vi "alignTop.vi"(6 "useControlBodyOnly":bool, 8 "error in (no error)":errorcluster, 11 "refs":refnum<vi>[](array[refnum])) -> (0 "error out":errorcluster, 3 "refs(dup)":refnum<vi>[](array[refnum]))   [LabVIEW 2023, in "TLC_Geometry.lvlib"]
doc: "Aligns all controls to the topmost position among the input controls.\nThe topmost coordinate is computed and applied to all controls."
uses:
  TLC_Geometry.lvlib
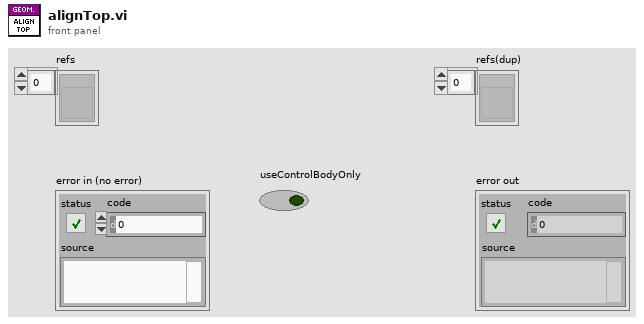
[diagram p1: front panel]
types:
  T1 = cluster{"left":i32, "top":i32, "right":i32, "bottom":i32}
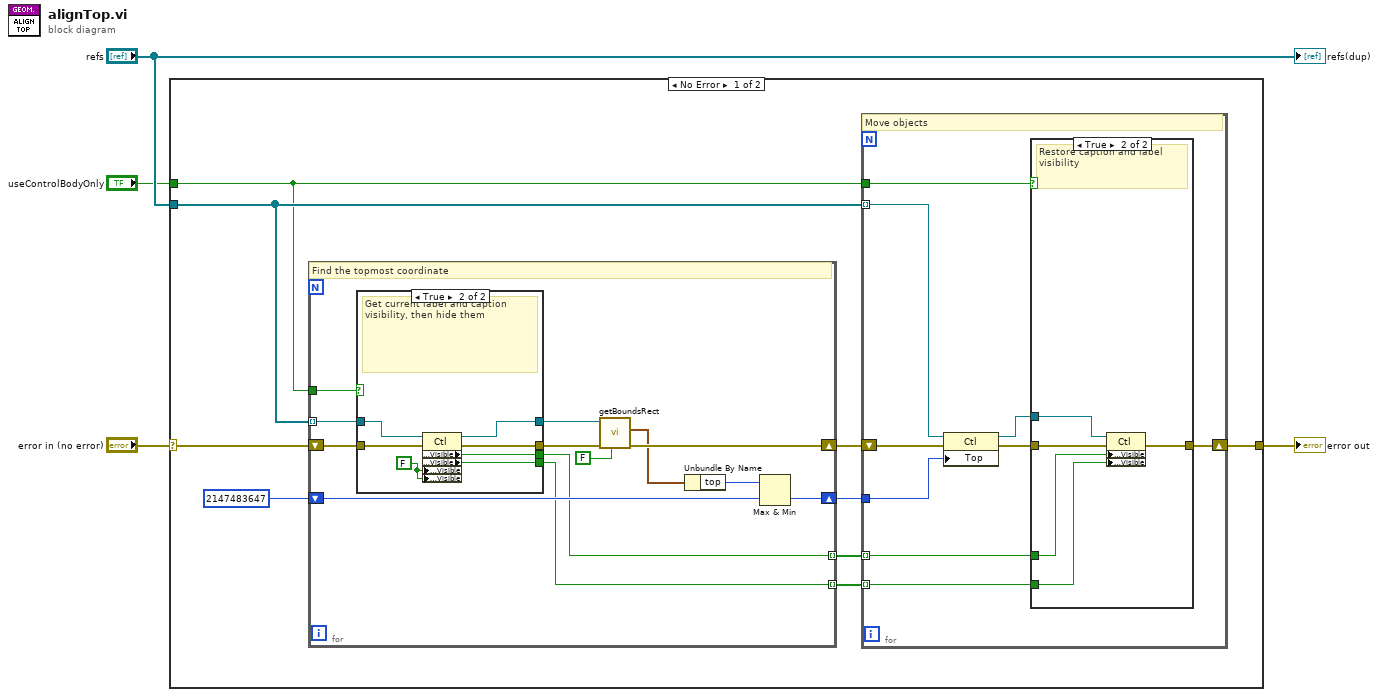
[diagram p0: block diagram]
diagram:
  n1 = case shown="No Error" "error in (no error)" {
    selector: "error in (no error)" -> [w13 w51]
    tunnel: [w10 w51] -> w1
    tunnel: "refs" -> [w11 _]
    tunnel: "useControlBodyOnly" -> [w7 _]
    frame No Error {
      n2 = for {
        tunnel: w11 -> [w36] mode=indexing
        shift-right: [w41] -> w9
        shift-left: w13 -> [w35]
        shift-right: [w30] -> w8
        shift-left: 2147483647 -> [w39]
        tunnel: w7 -> [w33]
        tunnel: [w32] -> w6 mode=indexing
        tunnel: [w31] -> w5 mode=indexing
        # "Find the topmost coordinate"
        n3 = case shown="True" w33 {
          tunnel: [w43 w50] -> w37
          tunnel: w36 -> [w43 w49]
          tunnel: w35 -> [w42 w48]
          tunnel: [w42 w47] -> w34
          tunnel: [_ w46] -> w32
          tunnel: [_ w45] -> w31
          frame False {
            # "Do nothing"
          }
          frame True {
            w44 = FALSE ("Caption.Visible")
            # "Get current label and caption visibility, then hide them"
            n4 = property class="Ctl"(reference=w49, error in=w48, "Caption.Visible"=w44, "Label.Visible"=w44) -> (reference out=w50:refnum<vi>, error out=w47:errorcluster, "Caption.Visible"=w46:bool, "Label.Visible"=w45:bool)
          }
        }
        n5 = call "getBoundsRect.vi"("ignoreCaption&Labels"=FALSE, "error in (no error)"=w34, "ref"=w37) -> ("error out"=w41:errorcluster, "rect"=w38:T1)  [unwired: 6 in, 1 out]
        n6 = Unbundle By Name(w38) -> ("top"=w40:i32)
        n7 = Max & Min(x=w40, y=w39) -> (min(x,y)=w30:i32)  [unwired: 1 out]
      }
      n8 = for {
        tunnel: w11 -> [w22] mode=indexing
        shift-right: [w19] -> w10
        shift-left: w9 -> [w20]
        tunnel: w8 -> [w21]
        tunnel: w7 -> [w17]
        tunnel: w6 -> [w15] mode=indexing
        tunnel: w5 -> [w14] mode=indexing
        # "Move objects"
        n9 = property class="Ctl"(reference=w22, error in=w20, "Top"=w21) -> (reference out=w16:refnum<vi>, error out=w18:errorcluster)
        n10 = case shown="True" w17 {
          tunnel: w16 -> [_ w28]
          tunnel: w18 -> [w23 w27]
          tunnel: [w23 w26] -> w19
          tunnel: w15 -> [_ w25]
          tunnel: w14 -> [_ w24]
          frame False {
            # "Do nothing"
          }
          frame True {
            # "Restore caption and label visibility"
            n11 = property class="Ctl"(reference=w28, error in=w27, "Caption.Visible"=w25, "Label.Visible"=w24) -> (error out=w26:errorcluster)  [unwired: 1 out]
          }
        }
      }
    }
    frame Error {
    }
  }
  "error out" <- w1
  "refs(dup)" <- "refs"
